vi "WeatherStationTester.vi"() -> ()   [LabVIEW 2012]
panel:
  out "AbsoluteHumidity":dbl
  out "Density":dbl
  out "Abs Humidity":dbl
  out "Coverted":dbl[](array[numeric])
  out "Raw":dbl[](array[numeric])
  out "Error Out":errorcluster
  in  "Error In":errorcluster
  in  "VISA in":refnum<visa-resource-name>="LuftWS"
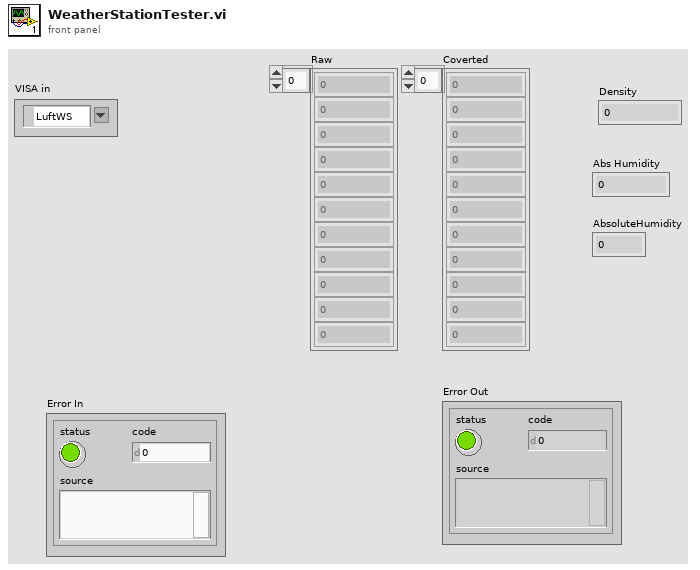
[diagram p1: front panel]
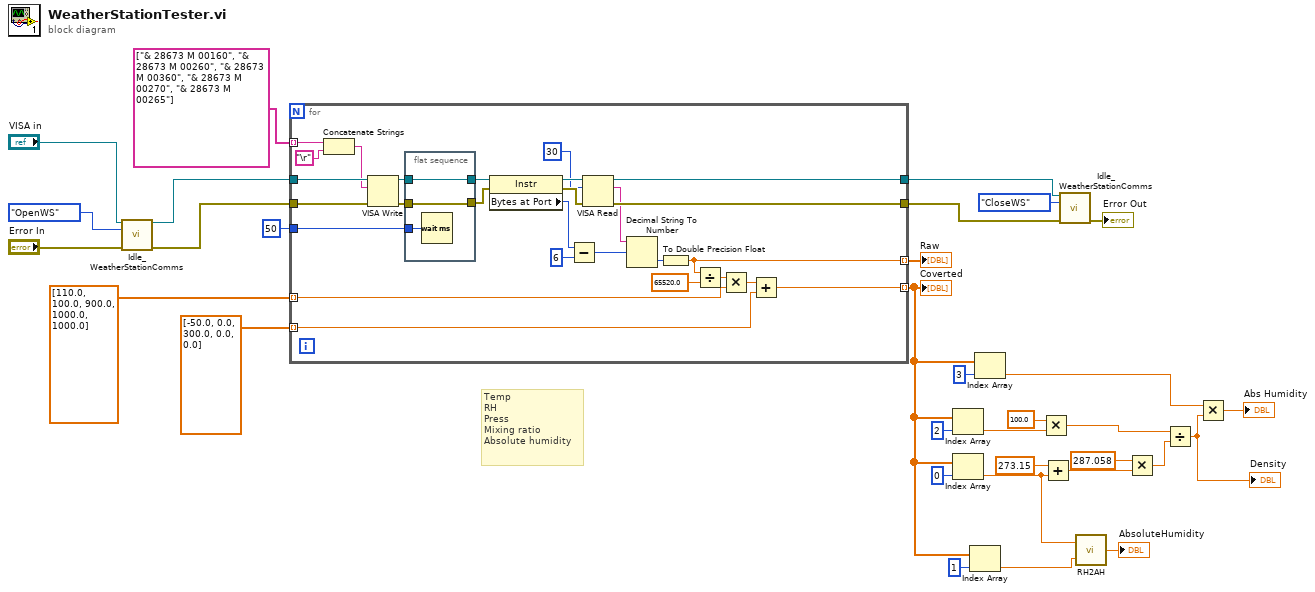
[diagram p0: block diagram]
diagram:
  # "Temp\nRH\nPress\nMixing ratio\nAbsolute humidity"
  n1 = call "Idle_WeatherStationComms.vi"("VISA in"="VISA in", "WS_Commands"=enum16{"OpenWS", "ReadTRHP", "CloseWS"}."OpenWS", "Error In"="Error In") -> ("VISA out"=w27:refnum<visa-resource-name>, "Error Out"=w26:errorcluster)  [unwired: 9 in, 2 out]
  n2 = for {
    tunnel: w27 -> [w59]
    tunnel: w26 -> [w58]
    tunnel: u32 50 ("wait (ms)") -> [w54]
    tunnel: [w49] -> w21
    tunnel: [w48] -> w20
    tunnel: [w34] -> w3 mode=indexing
    tunnel: string[] ["& 28673 M 00160", "& 28673 M 00260", "& 28673 M 00360", "& 28673 M 00270", "& 28673 M 00265"] -> [w38] mode=indexing
    tunnel: dbl[] [110.0, 100.0, 900.0, 1000.0, 1000.0] -> [w37] mode=indexing
    tunnel: dbl[] [-50.0, 0.0, 300.0, 0.0, 0.0] -> [w36] mode=indexing
    tunnel: [w33] -> w19 mode=indexing
    n3 = Concatenate Strings(w38, "\r") -> (w55:string)
    n4 = VISA Write(VISA resource name=w59, write buffer=w55, error in (no error)=w58) -> (VISA resource name out=w56:refnum<visa-resource-name>, error out=w57:errorcluster)  [unwired: 1 out]
    n5 = flat-sequence {
      tunnel: [w62] -> w51
      tunnel: w56 -> [w62]
      tunnel: [w61] -> w50
      tunnel: w57 -> [w61]
      tunnel: w54 -> [w60]
      frame #0 {
        n6 = Wait (ms)(milliseconds to wait=w60) -> ()  [unwired: 1 out]
      }
    }
    n7 = property class="Instr"(reference=w51, error in=w50) -> (reference out=w52:refnum<visa-resource-name>, error out=w53:errorcluster, "Bytes at Port"=w47:u32)
    n8 = Subtract(x=w47, y=u32 6) -> (x-y=w44:u32)
    n9 = VISA Read(VISA resource name=w52, byte count=u32 30, error in (no error)=w53) -> (VISA resource name out=w49:refnum<visa-resource-name>, read buffer=w45:string, error out=w48:errorcluster)  [unwired: 1 out]
    n10 = Decimal String To Number(string=w45, offset=w44) -> (number=w43:i32)  [unwired: 1 in, 1 out]
    n11 = To Double Precision Float(number=w43) -> (double precision float=w33:dbl)
    n12 = Divide(x=w33, y=65520.0) -> (x/y=w42:dbl)
    n13 = Multiply(x=w42, y=w37) -> (x*y=w41:dbl)
    n14 = Add(x=w41, y=w36) -> (x+y=w34:dbl)
  }
  "Raw" <- w19
  "Coverted" <- w3
  n15 = Index Array(array=w3, index=2) -> (element=w17:dbl)
  n16 = Index Array(array=w3, index=0) -> (element=w5:dbl)
  n17 = Index Array(array=w3, index=1) -> (element=w2:dbl)
  n18 = Index Array(array=w3, index=3) -> (element=w7:dbl)
  n19 = Multiply(x=100.0, y=w17) -> (x*y=w11:dbl)
  n20 = Add(x=273.15, y=w5) -> (x+y=w13:dbl)
  n21 = call "Idle_WeatherStationComms.vi"("VISA in"=w21, "WS_Commands"=enum16{"OpenWS", "ReadTRHP", "CloseWS"}."CloseWS", "Error In"=w20) -> ("Error Out"=→"Error Out":errorcluster)  [unwired: 9 in, 3 out]
  n22 = call "RH2AH.vi"("RelativeHUmidity"=w2, "Temperature [C]"=w5) -> ("AbsoluteHumidity"=→"AbsoluteHumidity":dbl)
  n23 = Multiply(x=287.058, y=w13) -> (x*y=w10:dbl)
  n24 = Divide(x=w11, y=w10) -> (x/y=w8:dbl)
  "Density" <- w8
  n25 = Multiply(x=w7, y=w8) -> (x*y=→"Abs Humidity":dbl)
